vi "Check if UUT already passed.vi"(8 "error in (no error)":errorcluster) -> (0 "error out":errorcluster, 2 "Stop button hit":bool, 3 "Passed?":bool)   [LabVIEW 2013]
uses:
  Main Support/Global 2.vi
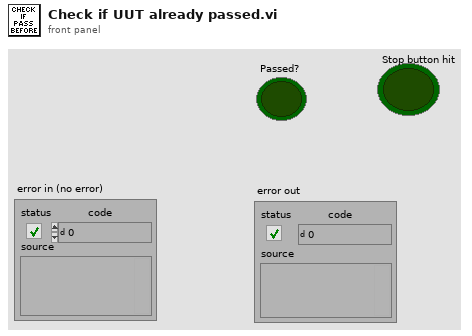
[diagram p1: front panel]
types:
  T1 = cluster{"Test folder":string, "Top level":string, "Main":string, "Test report":string, "Work order qty":string, "Work order meid":string, "Work order imei":string, "Master meid imei list":string, "Master test data":string, "ZPL label info":string, "Pictures":string, "Setup info":string, "Work order":string, "Tests folder":string, "Tests steps folder":string, "Config folder":string, "Verizon Upload file":string, "Job data file":string, "Station globals":string, "Post test info":string}
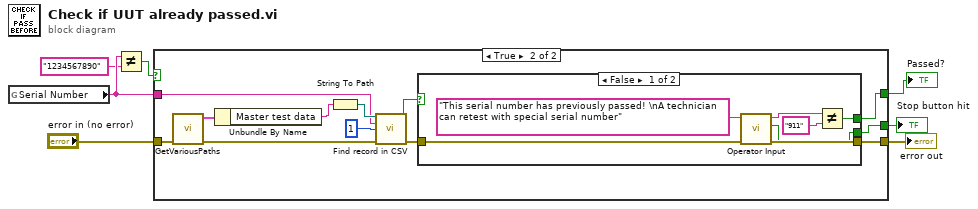
[diagram p0: block diagram]
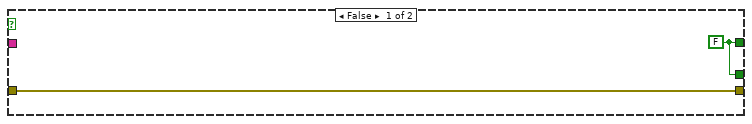
[diagram p2: hidden frame]
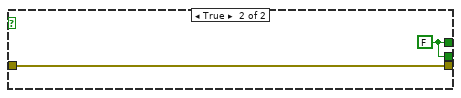
[diagram p3: hidden frame]
diagram:
  n1 = global read "Global 2.vi" "Serial Number"() -> (w4:string)
  n2 = Not Equal?(x=w4, y="1234567890") -> (x != y?=w2:bool)
  n3 = case shown="True" w2 {
    tunnel: [w8 w18] -> w7
    tunnel: "error in (no error)" -> [w9 w14]
    tunnel: [w9 w15] -> w5
    tunnel: w4 -> [_ w17]
    tunnel: [w8 w10] -> w1
    frame False {
      w8 = FALSE ("Passed?")
    }
    frame True {
      n4 = call "GetVariousPaths.vi"("error in (no error)"=w14) -> ("error out"=w13:errorcluster, "Built Paths"=w12:T1)  [unwired: 9 in]
      n5 = Unbundle By Name(w12) -> ("Master test data"=w11:string)
      n6 = String To Path(string=w11) -> (path=w20:path)
      n7 = call "Find record in CSV.vi"("CSV file"=w20, "Search key"=w17, "Search key column (0-n)"=u32 1, "error in"=w13) -> ("Record not found?"=w21:bool, "error out"=w16:errorcluster)  [unwired: 3 in, 7 out]
      n8 = case shown="False" w21 {
        tunnel: [w23 w29] -> w18
        tunnel: w16 -> [w27 w30]
        tunnel: [w26 w30] -> w15
        tunnel: [w22 w29] -> w10
        frame False {
          n9 = call "Operator Input.vi"("error in (no error)"=w27, "Message"="This serial number has previously passed! \nA technician can retest with special serial number" ("message")) -> ("error out"=w26:errorcluster, "Stop button hit"=w22:bool, "Response"=w25:string)  [unwired: 7 in]
          n10 = Not Equal?(x=w25, y="911") -> (x != y?=w23:bool)
        }
        frame True {
          w29 = FALSE ("Passed?")
        }
      }
    }
  }
  "Passed?" <- w7
  "error out" <- w5
  "Stop button hit" <- w1
